vi "rqp_Stop Listening.vi"(4 "Show in Debugger?":bool=TRUE, 6 "Message Priority":T1=enum."Normal", 7 "Caller in":refnum<class "Worker.lvclass">, 8 "error in":errorcluster, 11 "TCP Server in":refnum<class "TCP Server.lvclass">) -> (0 "error out":errorcluster, 3 "dup TCP Server out":refnum<class "TCP Server.lvclass">, 5 "dup Caller out":refnum<class "Worker.lvclass">)   [LabVIEW 2017, in "TCP Server.lvlib" / "TCP Server.lvclass"]
doc: "This VI sends a <b>Public API Request</b> message to an MHL case of the Worker that owns this VI.\n---\nStops the TCP Server from listening for any new connections from TCP Clients."
uses:
  TCP Server.lvclass
  C:/Program Files (x86)/National Instruments/LabVIEW 2017/vi.lib/addons/_Workers/Library/Classes/Worker/Worker.lvclass
  <vilib>/addons/_Workers/Library/Classes/Worker/Worker.lvclass
  <vilib>/addons/_Workers/Library/Classes/Message/Priority.ctl
  <vilib>/addons/_Workers/Library/Case Label.ctl
  rqp_Stop Listening.ctl
  <vilib>/addons/_Workers/Library/Classes/Message Queue/Message Queue.lvclass
  <vilib>/addons/_Workers/Library/Workers.lvlib
  <vilib>/addons/_Workers/Library/Classes/Message/Message.lvclass
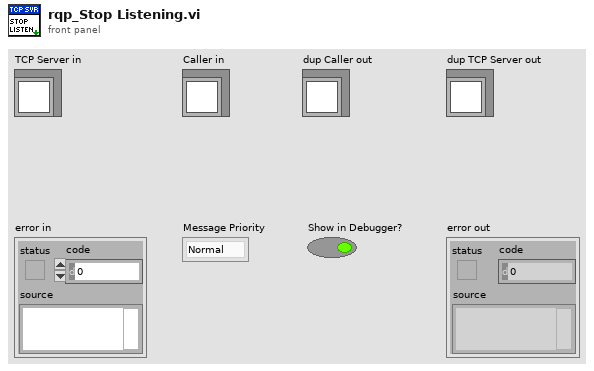
[diagram p1: front panel]
types:
  T1 = typedef "Workers.lvlib/Message.lvclass/Priority.ctl" = enum16{"Low", "Normal", "High"}
  T2 = typedef "TCP Server.lvlib/TCP Server.lvclass/rqp_Stop Listening.ctl" = cluster{"String":string}
  T3 = typedef "Workers.lvlib/Case Label.ctl" = string
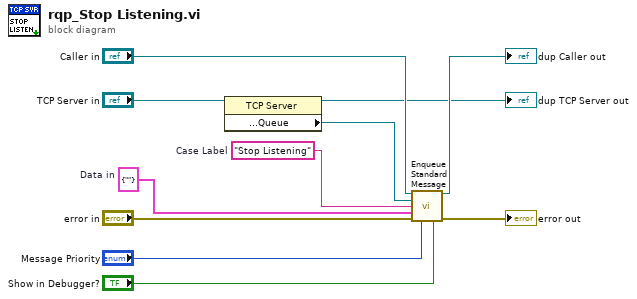
[diagram p0: block diagram]
diagram:
  w7 = T2 {"String"=""}  # Data in
  w1 = T3 "Stop Listening"  # Case Label
  n1 = property class="TCP Server"(reference="TCP Server in") -> (reference out=→"dup TCP Server out":refnum<class "TCP Server.lvclass">, "Accessors:Read:Public API:Queue"=w2:refnum<class "Message Queue.lvclass">)  [unwired: 1 in, 1 out]
  n2 = call-dynamic "Enqueue Standard Message.vi"("Worker"="Caller in", "Message Queue"=w2, "Case Label"=w1, "Data"=w7, "error in (no error)"="error in", "Priority (Normal)"="Message Priority", "Send Message to Debugger? (T)"="Show in Debugger?") -> ("dup Worker out"=→"dup Caller out":refnum<class "Worker.lvclass">, "error out"=→"error out":errorcluster)  [unwired: 7 in]
